vi "DIMPowerSupply.ProcDestructor.vi"(0 "i ref in":refnum<vi>, 5 "error in (no error)":errorcluster) -> (14 "i ref out":refnum<vi>, 19 "error out":errorcluster)   [LabVIEW 2014, in "DIMPowerSupply.lvlib"]
doc: "This is the counterpart to ProcConstructor and is called befor the \"deactivate\" is called. This can be used to shutdown/deinitialize things."
uses:
  DIMPowerSupply.lvlib
  CSlibraries-extern/DimLVEvent/LVDimInterface/LVDimInterface.lvlib
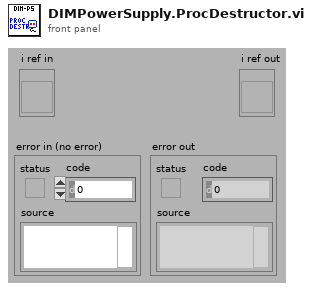
[diagram p1: front panel]
types:
  T1 = typedef "DIMPowerSupply.lvlib/DIMPowerSupply.i attribute.ctl" = cluster{"ctrlValueID":i32}
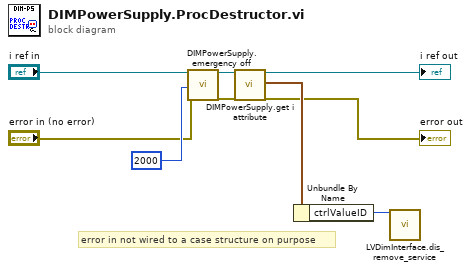
[diagram p0: block diagram]
diagram:
  # "error in not wired to a case structure on purpose"
  n1 = call "DIMPowerSupply.emergency off.vi"("i ref in"="i ref in", "ms timeout (10000)"=2000 ("ms timeout (100)"), "error in (no error)"="error in (no error)") -> ("i ref out"=w4:refnum<vi>, "error out"=w3:errorcluster)  [unwired: 14 in, 1 out]
  n2 = call "DIMPowerSupply.get i attribute.vi"("i ref in"=w4, "error in (no error)"=w3) -> ("i ref out"=→"i ref out":refnum<vi>, "i attribute"=w8:T1, "error out"=→"error out":errorcluster)  [unwired: 15 in]
  n3 = Unbundle By Name(w8) -> ("ctrlValueID"=w7:i32)
  n4 = call "LVDimInterface.dis_remove_service.vi"("my_serviceID"=w7) -> ()  [unwired: 18 in, 1 out]
